vi "Event Handle Loop_Mouse Leave.vi"(8 "error in (no error)":errorcluster, 11 "QMenu Class in":refnum<class "QMenu Class.lvclass">) -> (0 "error out":errorcluster, 3 "QMenu Class out":refnum<class "QMenu Class.lvclass">)   [LabVIEW 2020, in "QTab.lvlib" / "QMenu Class.lvclass"]
uses:
  QMenu Class.lvclass
  QMenu Class.lvclass/QMenu Class.ctl
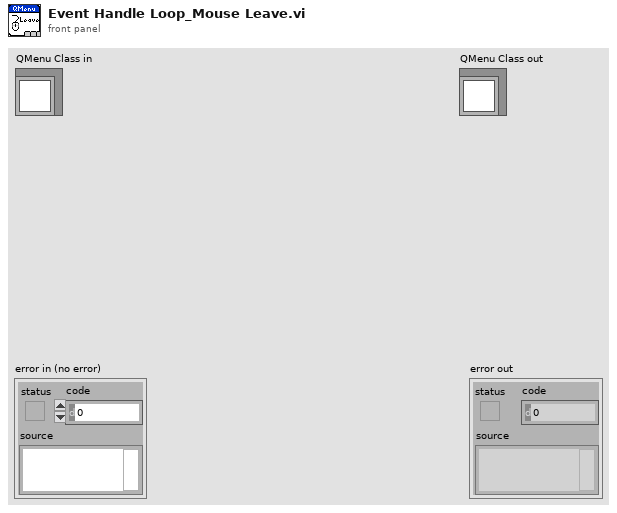
[diagram p1: front panel]
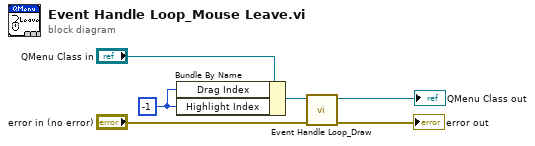
[diagram p0: block diagram]
diagram:
  w1 = -1 ("Focus Index")
  n1 = Bundle By Name(cluster="QMenu Class in", "Drag Index"=w1, "Highlight Index"=w1) -> (w2:refnum<class "QMenu Class.lvclass">)
  n2 = call "Event Handle Loop_Draw.vi"("error in (no error)"="error in (no error)", "QMenu Class in"=w2) -> ("error out"=→"error out":errorcluster, "QMenu Class out"=→"QMenu Class out":refnum<class "QMenu Class.lvclass">)  [unwired: 8 in]
